vi "Get Sub Objects.vi"(8 "error in":errorcluster, 11 "Obj Entry in":refnum<class "Object Entry.lvclass">) -> (0 "error out":errorcluster, 2 "Sub Objects":refnum<class "Sub Object.lvclass">[](array[class]), 3 "Obj Entry out":refnum<class "Object Entry.lvclass">)   [LabVIEW 2020, in "CANopen.lvlib" / "Object Entry.lvclass"]
uses:
  Object Entry.lvclass
  Object Entry.lvclass/Object Entry.ctl
  Sub Objects Dictionary/Sub Objects Dictionary.lvclass
  Sub Object/Sub Object.lvclass
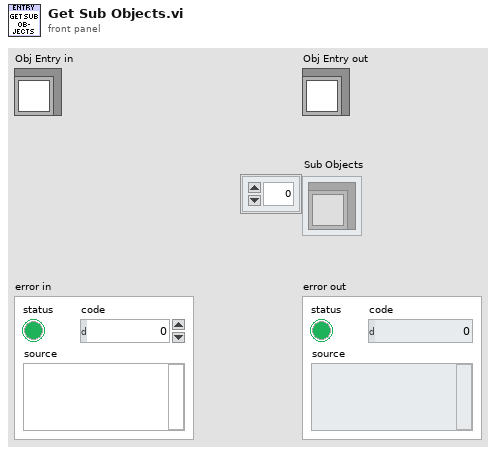
[diagram p1: front panel]
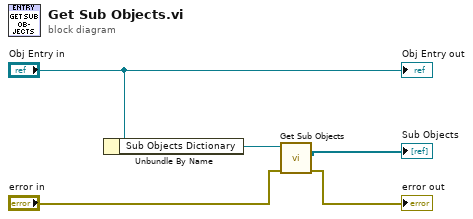
[diagram p0: block diagram]
diagram:
  n1 = Unbundle By Name("Obj Entry in") -> ("Sub Objects Dictionary"=w4:refnum<class "Sub Objects Dictionary.lvclass">)
  n2 = call "Get Sub Objects.vi"("error in"="error in", "Sub Objects Dictionary in"=w4) -> ("error out"=→"error out":errorcluster, "Sub Objects"=→"Sub Objects":refnum<class "Sub Object.lvclass">[])  [unwired: 7 in, 1 out]
  "Obj Entry out" <- "Obj Entry in"
